vi "TempFlowsLabels.vi"(7 "LabVIEW Web Service Request":refnum<class "Web Request.lvclass">) -> (0 "FuelData":bool=TRUE, 1 "FuelsLabels":T1(array[cluster]), 2 "TempData":bool=TRUE, 3 "TempsLabels":T3(array[cluster]))   [LabVIEW 2017]
uses:
  <vilib>/wsapi/Web Request.lvclass
panel:
  in  "f_q":dbl[][](array[numeric])
  in  "f_q 2":dbl[][](array[numeric])
  in  "array 2":variant[](array[variant])
  in  "FuelLabels":T2
  in  "array":variant[](array[variant])
  in  "TempLables":T4
  in  "Array 5":dbl[][](array[numeric])
  in  "temp typedef":dbl[][](array[numeric])
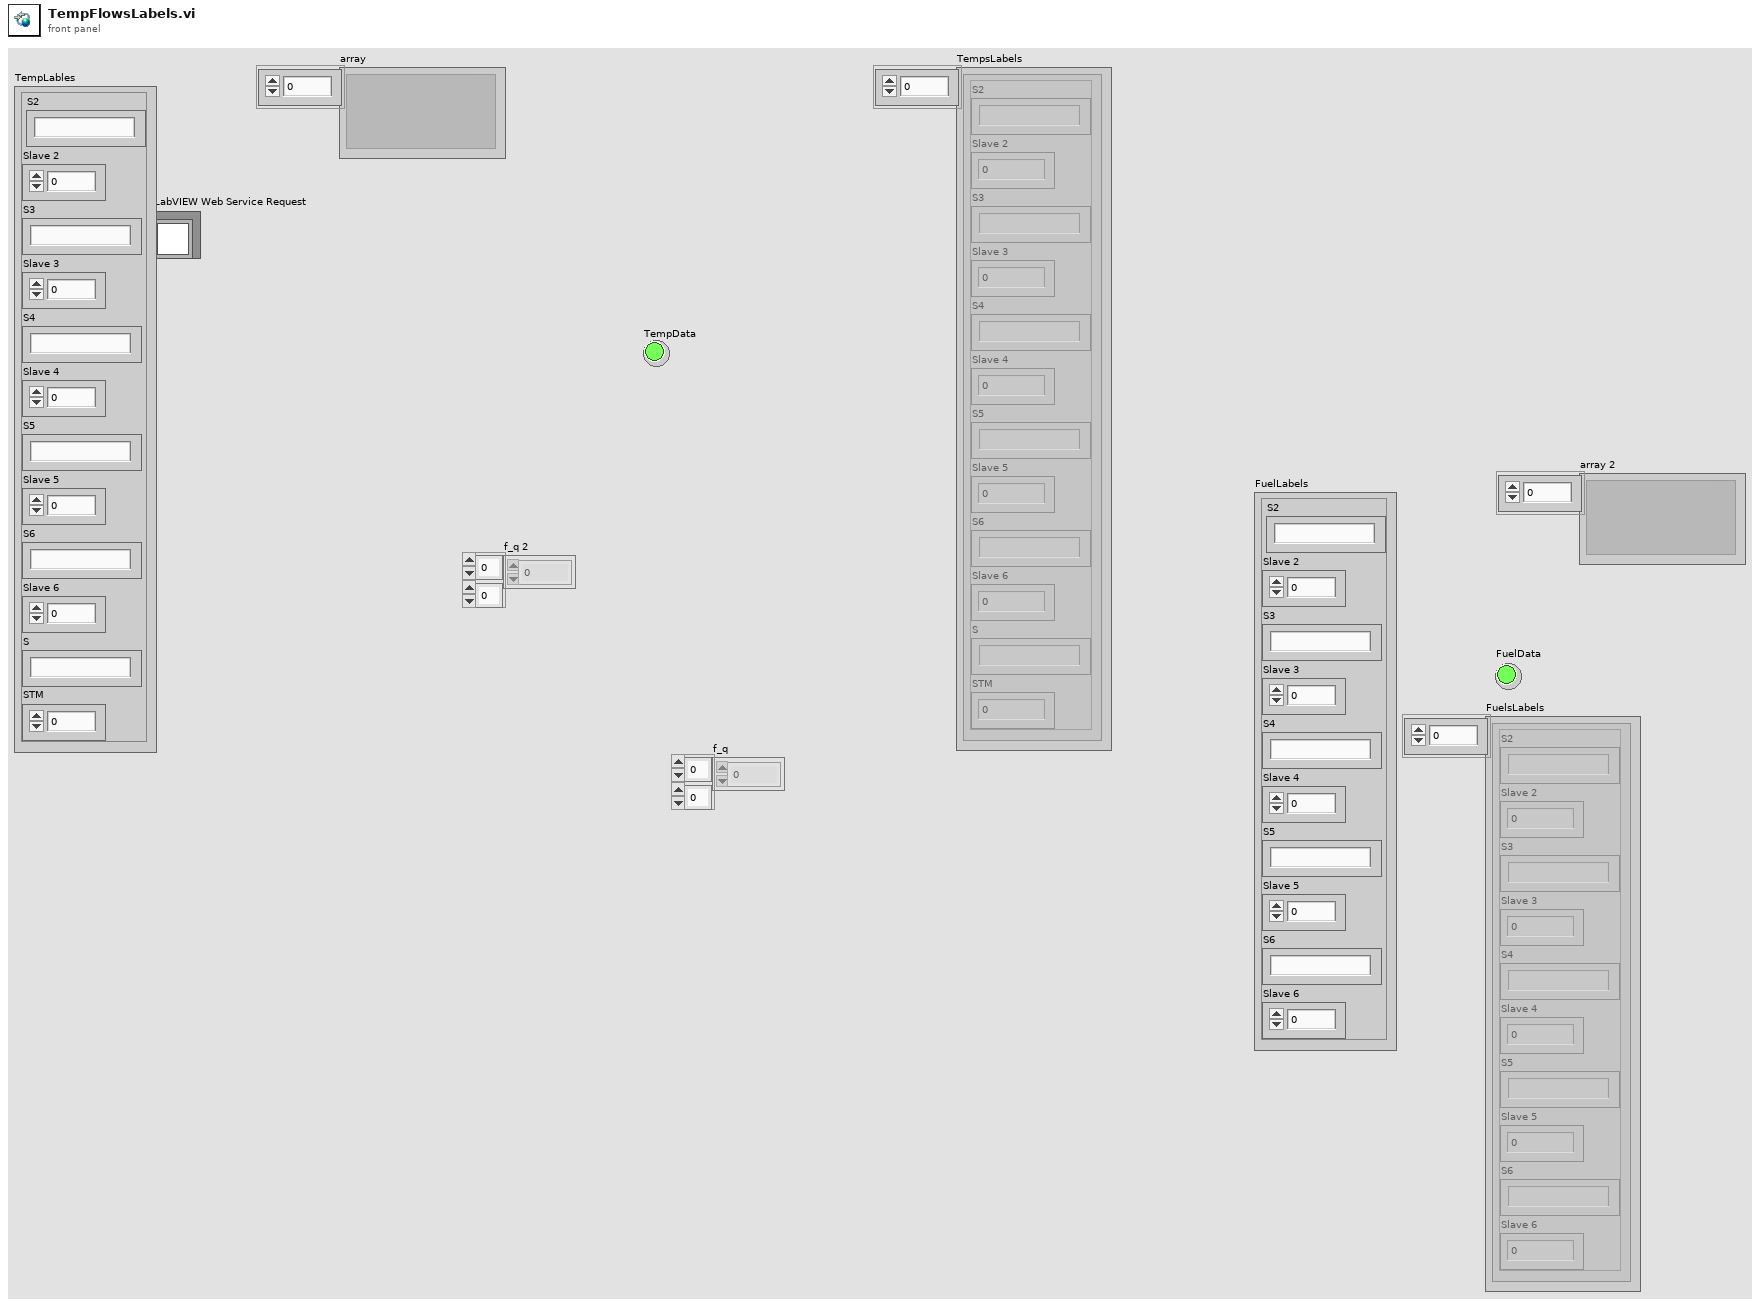
[diagram p1: front panel]
types:
  T1 = cluster{"S2":string, "Slave 2":dbl, "S3":string, "Slave 3":dbl, "S4":string, "Slave 4":dbl, "S5":string, "Slave 5":dbl, "S6":string, "Slave 6":dbl}[]
  T2 = cluster{"S2":string, "Slave 2":dbl, "S3":string, "Slave 3":dbl, "S4":string, "Slave 4":dbl, "S5":string, "Slave 5":dbl, "S6":string, "Slave 6":dbl}
  T3 = cluster{"S2":string, "Slave 2":dbl, "S3":string, "Slave 3":dbl, "S4":string, "Slave 4":dbl, "S5":string, "Slave 5":dbl, "S6":string, "Slave 6":dbl, "S":string, "STM":dbl}[]
  T4 = cluster{"S2":string, "Slave 2":dbl, "S3":string, "Slave 3":dbl, "S4":string, "Slave 4":dbl, "S5":string, "Slave 5":dbl, "S6":string, "Slave 6":dbl, "S":string, "STM":dbl}
  T5 = cluster{"Paliwo 1":string, "Paliwo 2":string, "Paliwo 3":string, "Paliwo 4":string, "Paliwo 5":string, "Paliwo 6":string}
  T6 = cluster{"Termometr 1":string, "Termometr 2":string, "Termometr 3":string, "Termometr 4":string, "Termometr 5":string, "Termometr 6":string, "Termometr 7":string, "Termometr 8":string, "Termometr 9":string, "Termometr 10":string}
  T7 = cluster{"array[0]":variant, "array[1]":variant, "array[2]":variant, "array[3]":variant, "array[4]":variant, "array[5]":variant, "array[6]":variant, "array[7]":variant, "array[8]":variant, "array[9]":variant, "array[10]":variant, "array[11]":variant}
  T8 = cluster{"array 2[0]":variant, "array 2[1]":variant, "array 2[2]":variant, "array 2[3]":variant, "array 2[4]":variant, "array 2[5]":variant, "array 2[6]":variant, "array 2[7]":variant, "array 2[8]":variant, "array 2[9]":variant}
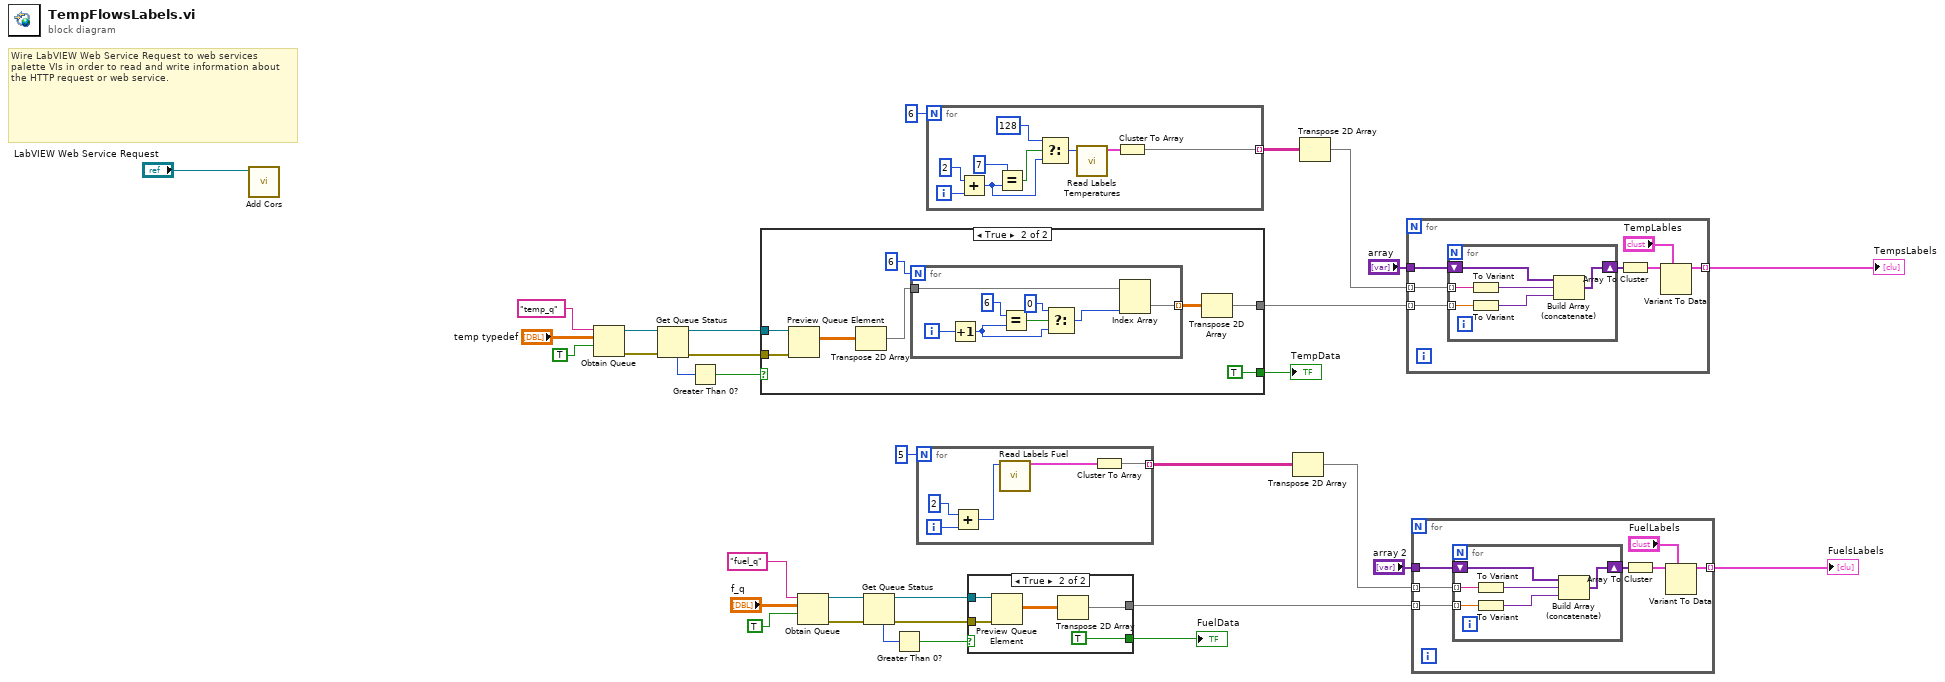
[diagram p0: block diagram]
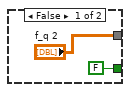
[diagram p2: hidden frame]
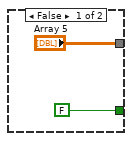
[diagram p3: hidden frame]
diagram:
  # "Wire LabVIEW Web Service Request to web services palette VIs in order to read and write information about the HTTP request or web service."
  n1 = call "Add Cors.vi"("Web Request in"="LabVIEW Web Service Request") -> ()  [unwired: 10 in, 1 out]
  n2 = Obtain Queue(name (unnamed)="temp_q", element data type="temp typedef", create if not found? (T)=TRUE) -> (queue out=w25:refnum<queue>, error out=w26:errorcluster)  [unwired: 2 in, 1 out]
  n3 = Get Queue Status(queue=w25, error in (no error)=w26) -> (queue out=w31:refnum<queue>, error out=w32:errorcluster, # elements in queue=w33:i32)  [unwired: 1 in, 5 out]
  n4 = Greater Than 0?(x=w33) -> (x > 0?=w30:bool)
  n5 = case shown="True" w30 {
    tunnel: w32 -> [_ w42]
    tunnel: w31 -> [_ w43]
    tunnel: ["Array 5" w36] -> w20
    tunnel: [FALSE TRUE] -> w24
    frame False {
    }
    frame True {
      n6 = Preview Queue Element(queue=w43, error in (no error)=w42) -> (element=w40:dbl[][])  [unwired: 1 in, 3 out]
      n7 = Transpose 2D Array(2D array=w40) -> (transposed array=w38:dbl[][])
      n8 = for {
        N: 6 -> [_]
        tunnel: w38 -> [w50]
        tunnel: [w49] -> w37 mode=indexing
        i -> [w51]
        n9 = Increment(x=w51) -> (x+1=w44:i32)
        n10 = Equal?(x=6 ("y"), y=w44) -> (x = y?=w48:bool)
        n11 = Select(t=0, s=w48, f=w44) -> (s? t:f=w45:i32)
        n12 = Index Array(array=w50, index (col)=w45) -> (element=w49:dbl[])  [unwired: 1 in]
      }
      n13 = Transpose 2D Array(2D array=w37) -> (transposed array=w36:dbl[][])
    }
  }
  "TempData" <- w24
  n14 = Obtain Queue(name (unnamed)="fuel_q", element data type="f_q", create if not found? (T)=TRUE) -> (queue out=w6:refnum<queue>, error out=w5:errorcluster)  [unwired: 2 in, 1 out]
  n15 = Get Queue Status(queue=w6, error in (no error)=w5) -> (queue out=w9:refnum<queue>, error out=w10:errorcluster, # elements in queue=w12:i32)  [unwired: 1 in, 5 out]
  n16 = Greater Than 0?(x=w12) -> (x > 0?=w11:bool)
  n17 = for {
    N: 5 -> [_]
    tunnel: [w53] -> w15 mode=indexing
    i -> [w56]
    n18 = Add(x=2, y=w56) -> (x+y=w54:i32)
    n19 = call "Read Labels Fuel.vi"("Slave ID"=w54) -> ("Etykiety P1-6"=w52:T5)  [unwired: 10 in]
    n20 = Cluster To Array(cluster=w52) -> (array=w53:string[])
  }
  n21 = for {
    N: 6 -> [_]
    tunnel: [w57] -> w21 mode=indexing
    i -> [w65]
    n22 = Add(x=2, y=w65) -> (x+y=w60:i32)
    n23 = Equal?(x=7, y=w60) -> (x = y?=w61:bool)
    n24 = Select(t=128, s=w61, f=w60) -> (s? t:f=w63:i32)
    n25 = call "Read Labels Temperatures.vi"("Slave ID"=w63) -> ("Etykiety T1-10"=w58:T6)  [unwired: 10 in]
    n26 = Cluster To Array(cluster=w58) -> (array=w57:string[])
  }
  n27 = case shown="True" w11 {
    tunnel: w9 -> [_ w72]
    tunnel: w10 -> [_ w71]
    tunnel: ["f_q 2" w68] -> w3
    tunnel: [FALSE TRUE] -> w4
    frame False {
    }
    frame True {
      n28 = Preview Queue Element(queue=w72, error in (no error)=w71) -> (element=w69:dbl[][])  [unwired: 1 in, 3 out]
      n29 = Transpose 2D Array(2D array=w69) -> (transposed array=w68:dbl[][])
    }
  }
  "FuelData" <- w4
  n30 = Transpose 2D Array(2D array=w15) -> (transposed array=w13:string[][])
  n31 = Transpose 2D Array(2D array=w21) -> (transposed array=w19:string[][])
  n32 = for {
    tunnel: w20 -> [w78] mode=indexing
    tunnel: w19 -> [w79] mode=indexing
    tunnel: "array" -> [w77]
    tunnel: [w73] -> w17 mode=indexing
    n33 = for {
      tunnel: w79 -> [w84] mode=indexing
      tunnel: w78 -> [w85] mode=indexing
      shift-right: [w82] -> w76
      shift-left: w77 -> [w83]
      n34 = To Variant(anything=w84) -> (Variant=w81:variant)
      n35 = To Variant(anything=w85) -> (Variant=w80:variant)
      n36 = Build Array (concatenate)(w83, w81, w80) -> (w82:variant[])
    }
    n37 = Array To Cluster(array=w76) -> (cluster=w75:T7)
    n38 = Variant To Data(type="TempLables", Variant=w75) -> (data=w73:T4)  [unwired: 1 in, 1 out]
  }
  "TempsLabels" <- w17
  n39 = for {
    tunnel: w3 -> [w91] mode=indexing
    tunnel: w13 -> [w92] mode=indexing
    tunnel: "array 2" -> [w90]
    tunnel: [w86] -> w1 mode=indexing
    n40 = for {
      tunnel: w92 -> [w97] mode=indexing
      tunnel: w91 -> [w98] mode=indexing
      shift-right: [w95] -> w89
      shift-left: w90 -> [w96]
      n41 = To Variant(anything=w97) -> (Variant=w94:variant)
      n42 = To Variant(anything=w98) -> (Variant=w93:variant)
      n43 = Build Array (concatenate)(w96, w94, w93) -> (w95:variant[])
    }
    n44 = Array To Cluster(array=w89) -> (cluster=w88:T8)
    n45 = Variant To Data(type="FuelLabels", Variant=w88) -> (data=w86:T2)  [unwired: 1 in, 1 out]
  }
  "FuelsLabels" <- w1
